vi "E36313A_Set_Volt_Curr.vi"(7 "Function (0 : Current)":i32(ring) items=["Current", "Voltage"], 8 "error in (no error)":errorcluster, 9 "Voltage Or Current Level (1)":dbl=1.0, 10 "Channel (1)":string="1", 11 "VISA resource name":refnum<visa-resource-name>) -> (0 "error out":errorcluster, 3 "VISA resource name out":refnum<visa-resource-name>)   [LabVIEW 2016]
uses:
  <instrlib>/Keysight E36300 Series/Keysight E36300 Series.lvlib
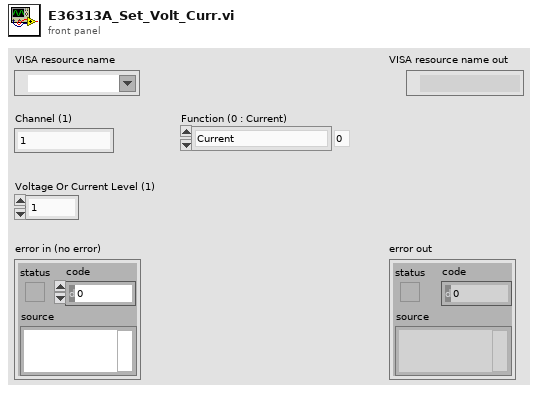
[diagram p1: front panel]
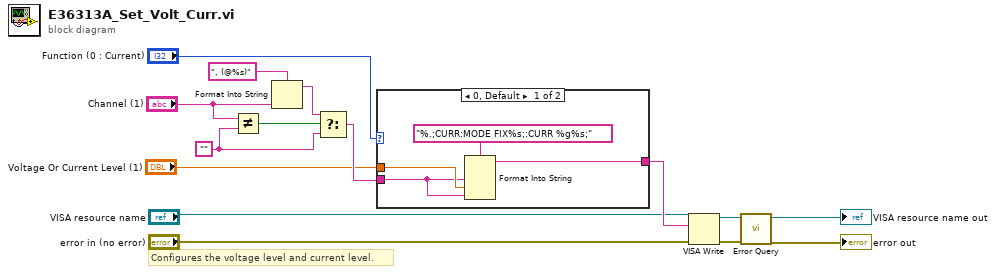
[diagram p0: block diagram]
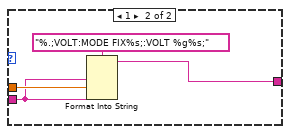
[diagram p2: hidden frame]
diagram:
  w15 = ""
  # "Configures the voltage level and current level."
  n1 = Not Equal?(x="Channel (1)", y=w15) -> (x != y?=w12:bool)
  n2 = Format Into String(format string=", (@%s)", "Channel (1)") -> (resulting string=w11:string)  [unwired: 2 in, 1 out]
  n3 = Select(t=w11, s=w12, f=w15) -> (s? t:f=w14:string)
  n4 = case shown="0, Default" "Function (0 : Current)" {
    tunnel: "Voltage Or Current Level (1)" -> [w18 w21]
    tunnel: [w17 w22] -> w9
    tunnel: w14 -> [w16 w20]
    frame 0, Default {
      n5 = Format Into String(format string="%.;CURR:MODE FIX%s;:CURR %g%s;", w16, w18, w16) -> (resulting string=w17:string)  [unwired: 2 in, 1 out]
    }
    frame 1 {
      n6 = Format Into String(format string="%.;VOLT:MODE FIX%s;:VOLT %g%s;", w20, w21, w20) -> (resulting string=w22:string)  [unwired: 2 in, 1 out]
    }
  }
  n7 = VISA Write(VISA resource name="VISA resource name", write buffer=w9, error in (no error)="error in (no error)") -> (VISA resource name out=w4:refnum<visa-resource-name>, error out=w5:errorcluster)  [unwired: 1 out]
  n8 = call <instrlib>:"Error Query.vi"("error in (no error)"=w5, "VISA resource name"=w4) -> ("error out"=→"error out":errorcluster, "VISA resource name out"=→"VISA resource name out":refnum<visa-resource-name>)  [unwired: 6 in, 2 out]
